vi "failUnlessXmlGeneratedCorrectly.vi"(4 "Convert EOL? (TRUE)":bool=TRUE, 6 "message (\"\")":string, 8 "error in":errorcluster, 9 "expected XML string":string, 10 "Input Data":variant, 11 "EasyXMLTest in":refnum<class "EasyXML_XML_Subset_Evaluations.lvclass">) -> (0 "error out":errorcluster, 2 "Generated XML String":string, 3 "EasyXMLTest out":refnum<class "EasyXML_XML_Subset_Evaluations.lvclass">)   [LabVIEW 2011, in "EasyXML_XML_Subset_Evaluations.lvclass"]
uses:
  EasyXML_XML_Subset_Evaluations.lvclass
panel:
  # "Copyright © 2007 James Kring, Inc. All rights reserved.\n\nAuthor: Jim Kring [jim.kring@jameskring.com]\n\nThis library is provided \"AS IS\" ,WITHOUT WARRANTIES OR \nCONDITIONS OF ANY KIND, either express or implied.\n\nJames Kring, Inc. -- http://www.jameskring.com"
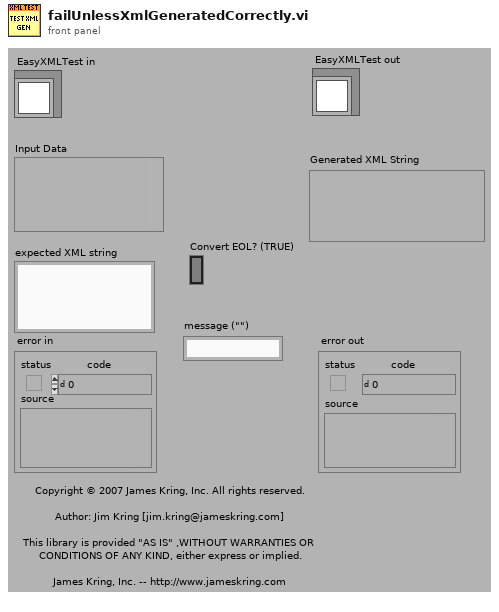
[diagram p1: front panel]
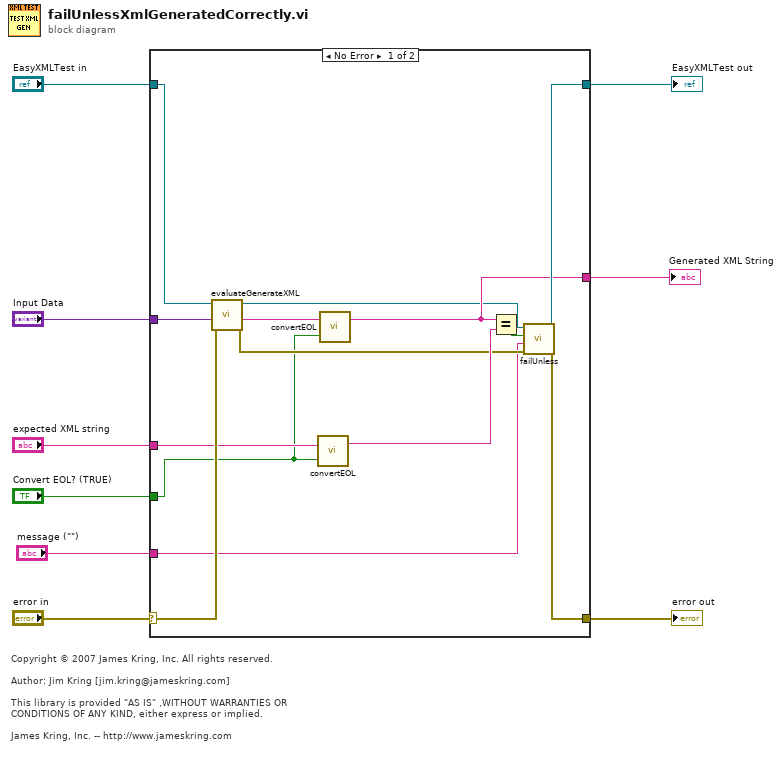
[diagram p0: block diagram]
diagram:
  # "Copyright © 2007 James Kring, Inc. All rights reserved.\n\nAuthor: Jim Kring [jim.kring@jameskring.com]\n\nThis library is provided \"AS IS\" ,WITHOUT WARRANTIES OR \nCONDITIONS OF ANY KIND, either express or implied.\n\nJames Kring, Inc. -- http://www.jameskring.com"
  n1 = case shown="No Error" "error in" {
    selector: "error in" -> [w22 w25]
    tunnel: [w18 w25] -> w4
    tunnel: "EasyXMLTest in" -> [w11 w24]
    tunnel: [w19 w24] -> w6
    tunnel: "Input Data" -> [w23 _]
    tunnel: "expected XML string" -> [w21 _]
    tunnel: "message (\"\")" -> [w15 _]
    tunnel: [w12 _] -> w2
    tunnel: "Convert EOL? (TRUE)" -> [w14 _]
    frame No Error {
      n2 = call-dynamic "evaluateGenerateXML.vi"("error in"=w22, "Input Data"=w23, "reference in"=w11) -> ("error out"=w17:errorcluster, "XML String"=w13:string, "reference out"=w10:refnum<class "EasyXML_XML_Subset_Evaluations.lvclass">)  [unwired: 6 in]
      n3 = call "convertEOL.vi"("Convert EOL? (TRUE)"=w14, "string"=w21) -> ("string out"=w20:string)  [unwired: 1 in]
      n4 = call "convertEOL.vi"("Convert EOL? (TRUE)"=w14, "string"=w13) -> ("string out"=w12:string)  [unwired: 1 in]
      n5 = Equal?(x=w12, y=w20) -> (x = y?=w16:bool)
      n6 = call-dynamic "failUnless.vi"("error in (no error)"=w17, "message (\"\")"=w15, "pass"=w16, "TestCase in"=w10) -> ("error out"=w18:errorcluster, "TestCase out"=w19:refnum<class "EasyXML_XML_Subset_Evaluations.lvclass">)  [unwired: 6 in]
    }
    frame Error {
    }
  }
  "EasyXMLTest out" <- w6
  "error out" <- w4
  "Generated XML String" <- w2
